vi "VI Tree.vi"   [LabVIEW 2022 SP3, in "Keithley 24XX.lvlib"]
doc: "This is the instrument driver for the Keithley 2400 Series SourceMeter. The VI Tree displays all the user-callable VIs of the instrument driver in an organized table."
uses:
  Keithley 24XX.lvlib
  Data/Read (Math).vi
  Data/Read (Statistical).vi
  Data/Read (Multiple Points).vi
  Data/Read (Single Point).vi
  Data/Low Level/Fetch (Measurements).vi
panel:
  # "(c) 2006 - 2015 National Instruments.  ALL RIGHTS RESERVED."
  # "SEE DIAGRAM\nFOR VI TREE."
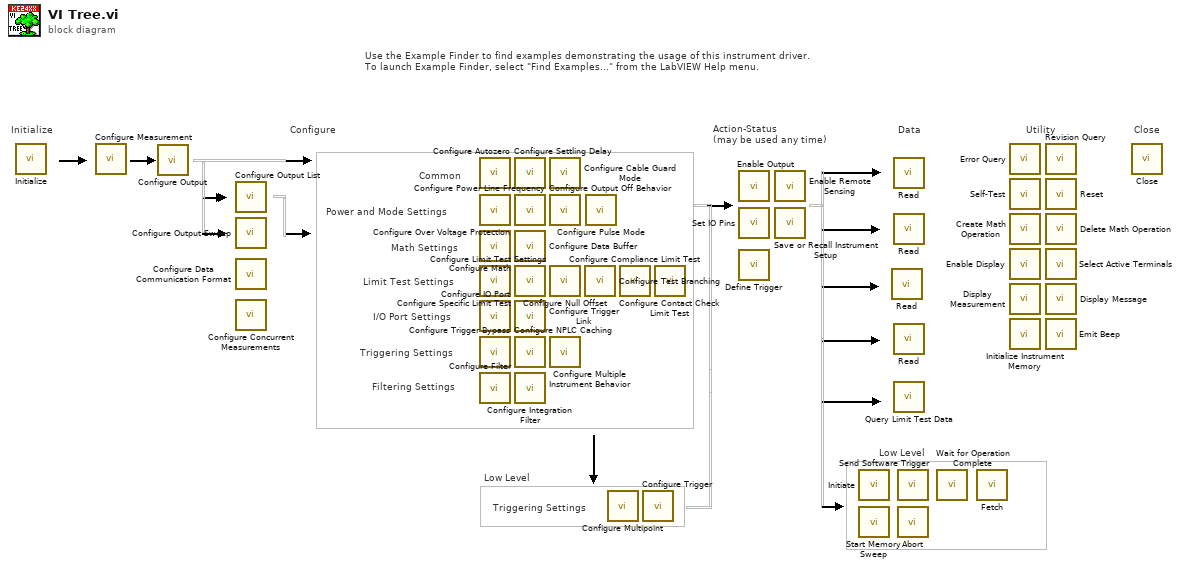
[diagram p0: block diagram]
diagram:
  # "Triggering Settings"
  # "Low Level"
  # "Action-Status\n(may be used any time)"
  # "Filtering Settings"
  # "Triggering Settings"
  # "Power and Mode Settings"
  # "Math Settings"
  # "Limit Test Settings"
  # "I/O Port Settings"
  # "Common"
  # "Low Level"
  # "Use the Example Finder to find examples demonstrating the usage of this instrument driver.\nTo launch Example Finder, select \"Find Examples...\" from the LabVIEW Help menu."
  # "Configure"
  # "Utility"
  # "Data"
  # "Close"
  # "Initialize"
  n1 = call "Initialize.vi"() -> ()  [unwired: 10 in, 2 out]
  n2 = call "Configure Measurement.vi"() -> ()  [unwired: 10 in, 2 out]
  n3 = call "Configure Output.vi"() -> ()  [unwired: 10 in, 2 out]
  n4 = call "Configure Output List.vi"() -> ()  [unwired: 10 in, 2 out]
  n5 = call "Configure Output Sweep.vi"() -> ()  [unwired: 14 in, 2 out]
  n6 = call "Configure Data Communication Format.vi"() -> ()  [unwired: 10 in, 2 out]
  n7 = call "Configure Concurrent Measurements.vi"() -> ()  [unwired: 10 in, 2 out]
  n8 = call "Configure Autozero.vi"() -> ()  [unwired: 10 in, 2 out]
  n9 = call "Configure Over Voltage Protection.vi"() -> ()  [unwired: 10 in, 2 out]
  n10 = call "Configure Math.vi"() -> ()  [unwired: 10 in, 2 out]
  n11 = call "Configure Specific Limit Test.vi"() -> ()  [unwired: 14 in, 2 out]
  n12 = call "Configure IO Port.vi"() -> ()  [unwired: 10 in, 2 out]
  n13 = call "Configure Trigger Bypass.vi"() -> ()  [unwired: 10 in, 2 out]
  n14 = call "Configure Filter.vi"() -> ()  [unwired: 10 in, 2 out]
  n15 = call "Configure Settling Delay.vi"() -> ()  [unwired: 10 in, 2 out]
  n16 = call "Configure Power Line Frequency.vi"() -> ()  [unwired: 10 in, 2 out]
  n17 = call "Configure Data Buffer.vi"() -> ()  [unwired: 10 in, 2 out]
  n18 = call "Configure Limit Test Settings.vi"() -> ()  [unwired: 10 in, 2 out]
  n19 = call "Configure Trigger Link.vi"() -> ()  [unwired: 14 in, 2 out]
  n20 = call "Configure NPLC Caching.vi"() -> ()  [unwired: 10 in, 2 out]
  n21 = call "Configure Integration Filter.vi"() -> ()  [unwired: 10 in, 2 out]
  n22 = call "Configure Cable Guard Mode.vi"() -> ()  [unwired: 10 in, 2 out]
  n23 = call "Configure Output Off Behavior.vi"() -> ()  [unwired: 10 in, 2 out]
  n24 = call "Configure Null Offset.vi"() -> ()  [unwired: 10 in, 2 out]
  n25 = call "Configure Multiple Instrument Behavior.vi"() -> ()  [unwired: 10 in, 2 out]
  n26 = call "Configure Test Branching.vi"() -> ()  [unwired: 10 in, 2 out]
  n27 = call "Configure Pulse Mode.vi"() -> ()  [unwired: 10 in, 2 out]
  n28 = call "Configure Multipoint.vi"() -> ()  [unwired: 10 in, 2 out]
  n29 = call "Configure Compliance Limit Test.vi"() -> ()  [unwired: 10 in, 2 out]
  n30 = call "Configure Trigger.vi"() -> ()  [unwired: 10 in, 2 out]
  n31 = call "Configure Contact Check Limit Test.vi"() -> ()  [unwired: 10 in, 2 out]
  n32 = call "Enable Output.vi"() -> ()  [unwired: 10 in, 2 out]
  n33 = call "Set IO Pins.vi"() -> ()  [unwired: 10 in, 2 out]
  n34 = call "Define Trigger.vi"() -> ()  [unwired: 10 in, 2 out]
  n35 = call "Enable Remote Sensing.vi"() -> ()  [unwired: 10 in, 2 out]
  n36 = call "Save or Recall Instrument Setup.vi"() -> ()  [unwired: 10 in, 2 out]
  n37 = call "Initiate.vi"() -> ()  [unwired: 10 in, 2 out]
  n38 = call "Start Memory Sweep.vi"() -> ()  [unwired: 10 in, 2 out]
  n39 = call-poly "Read.vi"() -> ()  [unwired: 13 in, 3 out]
  n40 = call-poly "Read.vi"() -> ()  [unwired: 9 in, 7 out]
  n41 = call-poly "Read.vi"() -> ()  [unwired: 9 in, 7 out]
  n42 = call-poly "Read.vi"() -> ()  [unwired: 13 in, 3 out]
  n43 = call "Query Limit Test Data.vi"() -> ()  [unwired: 9 in, 3 out]
  n44 = call "Send Software Trigger.vi"() -> ()  [unwired: 10 in, 2 out]
  n45 = call "Abort.vi"() -> ()  [unwired: 10 in, 2 out]
  n46 = call "Wait for Operation Complete.vi"() -> ()  [unwired: 10 in, 2 out]
  n47 = call-poly "Fetch.vi"() -> ()  [unwired: 9 in, 7 out]
  n48 = call "Error Query.vi"() -> ()  [unwired: 8 in, 4 out]
  n49 = call "Self-Test.vi"() -> ()  [unwired: 8 in, 4 out]
  n50 = call "Create Math Operation.vi"() -> ()  [unwired: 10 in, 2 out]
  n51 = call "Enable Display.vi"() -> ()  [unwired: 10 in, 2 out]
  n52 = call "Display Measurement.vi"() -> ()  [unwired: 10 in, 2 out]
  n53 = call "Initialize Instrument Memory.vi"() -> ()  [unwired: 10 in, 2 out]
  n54 = call "Revision Query.vi"() -> ()  [unwired: 8 in, 4 out]
  n55 = call "Reset.vi"() -> ()  [unwired: 10 in, 2 out]
  n56 = call "Delete Math Operation.vi"() -> ()  [unwired: 10 in, 2 out]
  n57 = call "Select Active Terminals.vi"() -> ()  [unwired: 10 in, 2 out]
  n58 = call "Display Message.vi"() -> ()  [unwired: 10 in, 2 out]
  n59 = call "Emit Beep.vi"() -> ()  [unwired: 10 in, 2 out]
  n60 = call "Close.vi"() -> ()  [unwired: 11 in, 1 out]
